vi "BPSK_DeModulation.vi"(4 "input_data":cdb[](array[numeric]), 5 ",EN_Modulation":dbl, 6 "ini_pha":dbl, 7 "y":dbl[](array[numeric]), 8 "error in (no error)":errorcluster caption="错误输入（无错误）", 11 "PathIn":path) -> (0 "error out":errorcluster caption="错误输出", 2 "re_data":dbl[](array[numeric]), 3 "PathOut":path)   [LabVIEW 2015]
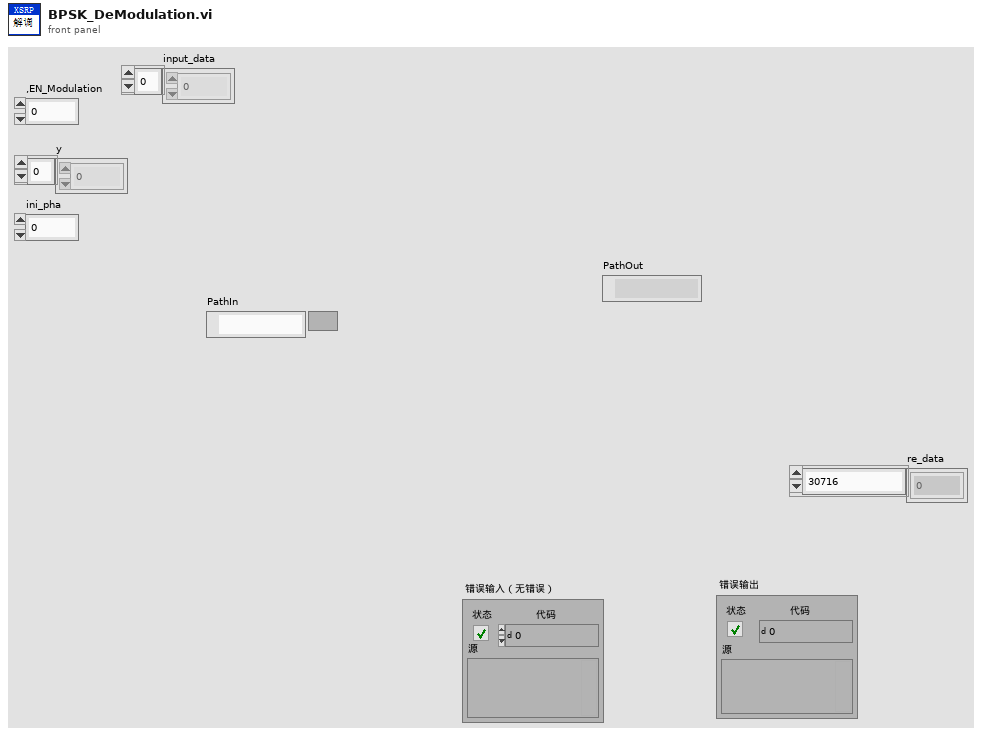
[diagram p1: front panel]
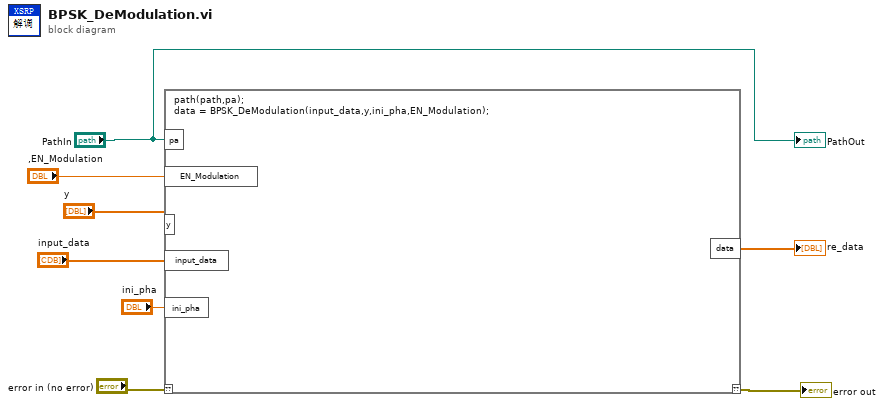
[diagram p0: block diagram]
diagram:
  n1 = script code="path(path,pa);\ndata = BPSK_DeModulation(input_data,y,ini_pha,EN_Modulation);"("??"="error in (no error)", "pa"="PathIn", "input_data"="input_data", "y"="y", "ini_pha"="ini_pha", "EN_Modulation"=",EN_Modulation") -> ("??"=→"error out":errorcluster, "data"=→"re_data":dbl[])
  "PathOut" <- "PathIn"
